vi "Switch_heater_wait.vi"(1 "T-Start":timestamp, 2 "Switch waiting time":dbl format="%#_13g") -> ()   [LabVIEW 2016]
uses:
  Global/Global Variables/Data_Display_global.vi
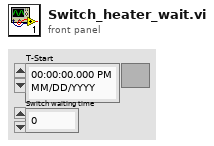
[diagram p1: front panel]
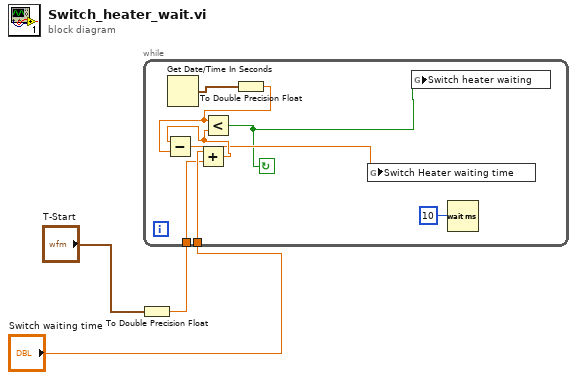
[diagram p0: block diagram]
diagram:
  n1 = To Double Precision Float(number="T-Start") -> (double precision float=w3:dbl)
  n2 = while {
    tunnel: "Switch waiting time" -> [w11]
    tunnel: w3 -> [w10]
    stop <- w7 continue-if-true
    n3 = Get Date/Time In Seconds() -> (seconds since 1Jan1904=w6:timestamp)
    n4 = Add(x=w11, y=w10) -> (x+y=w9:dbl)
    n5 = To Double Precision Float(number=w6) -> (double precision float=w5:dbl)
    n6 = Subtract(x=w9, y=w5) -> (x-y=w8:dbl)
    n7 = Less?(x=w5, y=w9) -> (x < y?=w7:bool)
    n8 = global write "Data_Display_global.vi" "Switch Heater waiting time"(w8) -> ()
    n9 = global write "Data_Display_global.vi" "Switch heater waiting"(w7) -> ()
    n10 = Wait (ms)(milliseconds to wait=10) -> ()  [unwired: 1 out]
  }
